vi "Interpolate and Measure.vi"(8 "error in (no error)":errorcluster, 9 "search results":cluster{"level":dbl, "value":dbl}[](array[cluster]), 10 "frequency (Hz)":dbl, 11 "measurement configuration":T2 {"acq sampling rate" format="%0.2f"; "master clock rate" format="%#_6pHz"; "frame clock rate" format="%#_6pHz"}) -> (0 "error out":errorcluster, 1 "spectrum":cluster{"x0":dbl, "dx":dbl, "magnitude":dbl[]}, 2 "time domain":waveform(dbl), 3 "results":T1, 4 "output power":dbl)   [LabVIEW 2021]
uses:
  Measurement Configuration.ctl
  shared/controls/digital audio protocol/data justification.ctl
  shared/controls/digital audio protocol/endianness.ctl
  shared/controls/digital audio protocol/digital edge.ctl
  shared/controls/digital audio protocol/logic level.ctl
  shared/controls/digital output level units.ctl
  shared/controls/weighting filter.ctl
  shared/controls/highpass filter.ctl
  shared/controls/lowpass filter.ctl
  shared/controls/sweep profile.ctl
  shared/controls/units - snr.ctl
  shared/controls/units - ratio.ctl
  shared/controls/regulation target.ctl
  shared/controls/regulation target value units.ctl
  Stepped Frequency Sweep_Class D Amplifier.lvlib
  <vilib>/Analysis/NI_AALPro.lvlib
  shared/controls/audio controls.lvlib
  shared/controls/single tone audio measurements.ctl
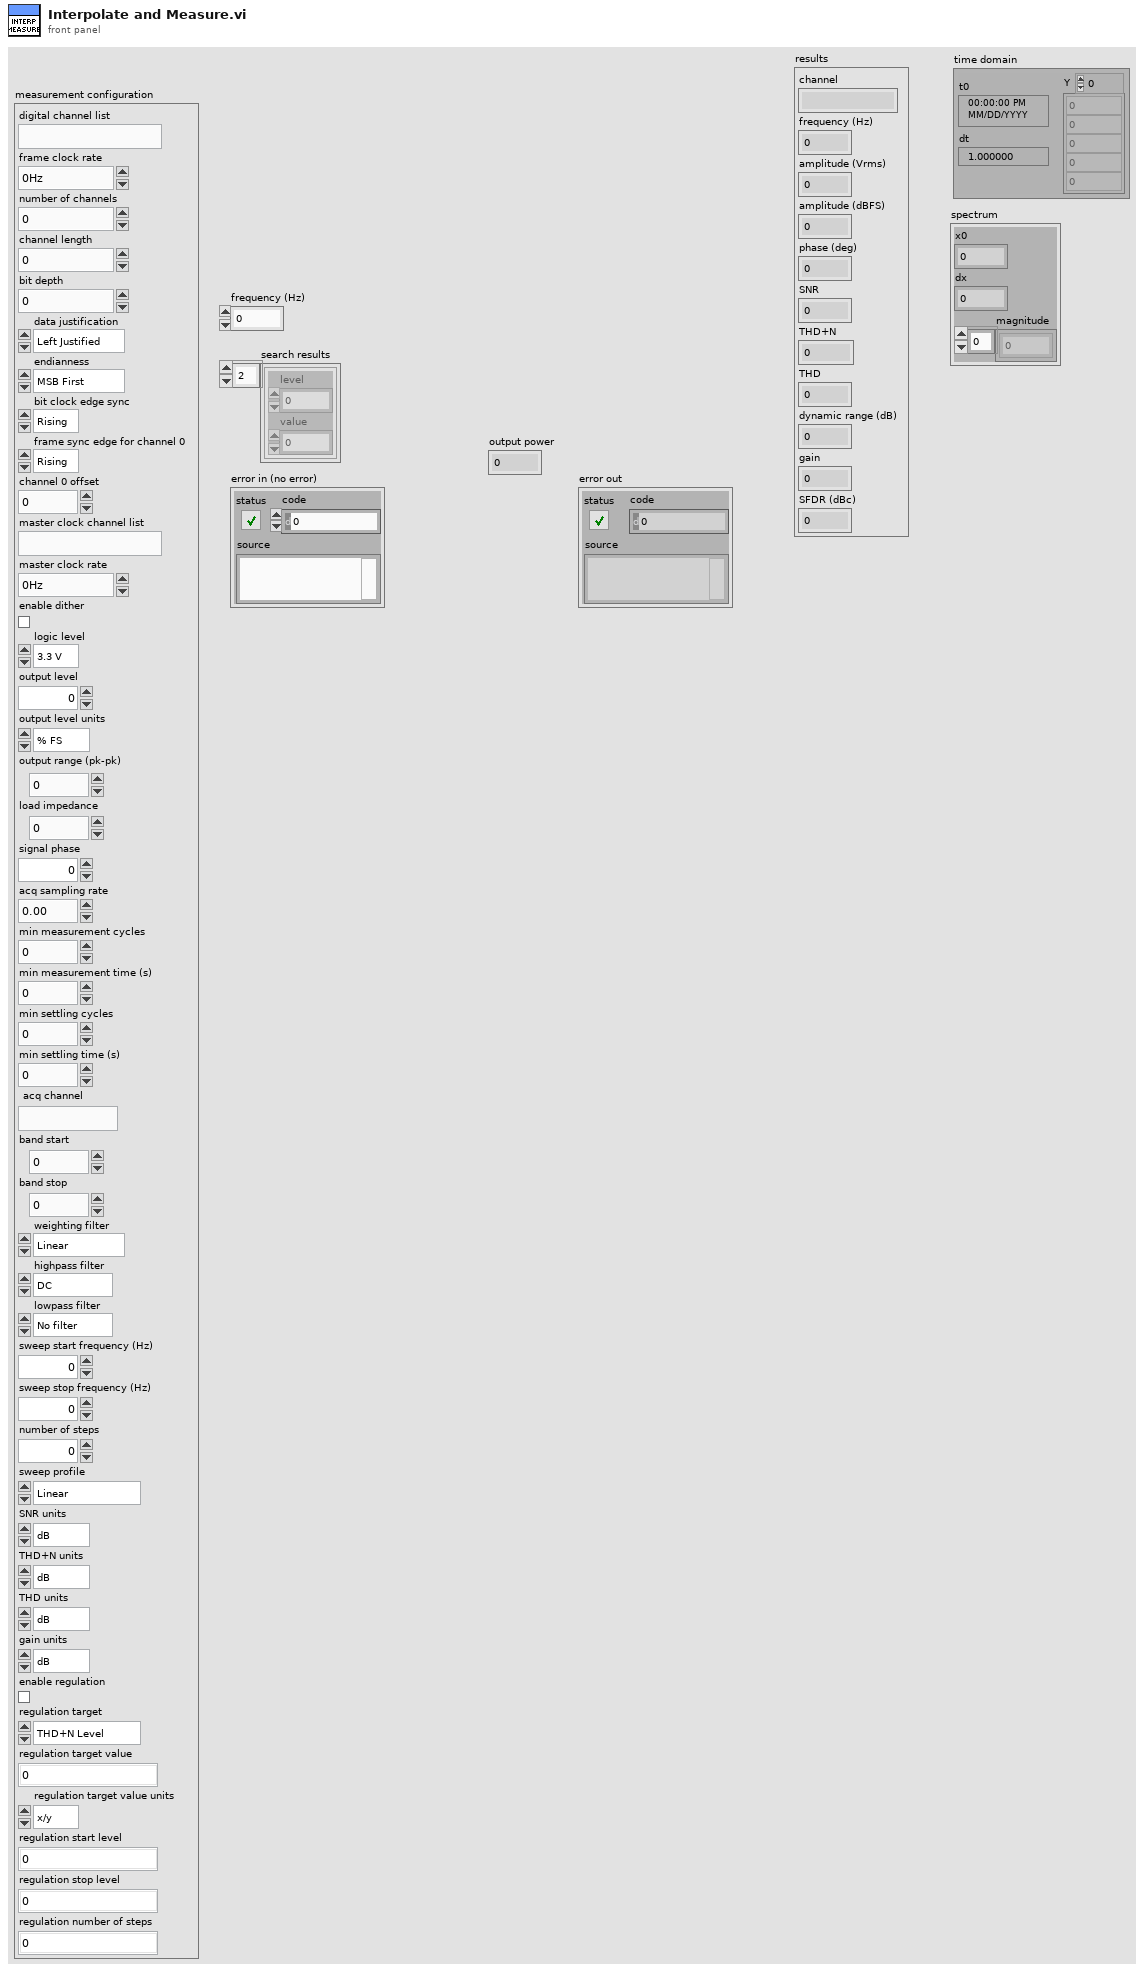
[diagram p1: front panel]
types:
  T1 = typedef "audio controls.lvlib/single tone audio measurements.ctl" = cluster{"channel":string, "frequency (Hz)":dbl, "amplitude (Vrms)":dbl, "amplitude (dBFS)":dbl, "phase (deg)":dbl, "SNR":dbl, "THD+N":dbl, "THD":dbl, "dynamic range (dB)":dbl, "gain":dbl, "SFDR (dBc)":dbl}
  T2 = typedef "Stepped Frequency Sweep_Class D Amplifier.lvlib/Measurement Configuration.ctl" = cluster{"digital channel list":string, "frame clock rate":dbl, "number of channels":u32, "channel length":u32, "bit depth":u32, "data justification":T3, "endianness":T4, "bit clock edge sync":T5, "frame sync edge for channel 0":T5, "channel 0 offset":u32, "master clock channel list":string, "master clock rate":dbl, "enable dither":bool, "logic level":T6, "output level":dbl, "output level units":T7, "output range (pk-pk)":dbl, "load impedance":dbl, "signal phase":dbl, "acq sampling rate":dbl, "min measurement cycles":u32, "min measurement time (s)":dbl, "min settling cycles":u32, "min settling time (s)":dbl, "acq channel":string, "band start":dbl, "band stop":dbl, "weighting filter":T8, "highpass filter":T9, "lowpass filter":T10, "sweep start frequency (Hz)":dbl, "sweep stop frequency (Hz)":dbl, "number of steps":u32, "sweep profile":T11, "SNR units":T12, "THD+N units":T13, "THD units":T13, "gain units":T13, "enable regulation":bool, "regulation target":T14, "regulation target value":dbl, "regulation target value units":T15, "regulation start level":dbl, "regulation stop level":dbl, "regulation number of steps":u32}
  T3 = typedef "data justification.ctl" = enum32{"Left Justified", "Right Justified"}
  T4 = typedef "endianness.ctl" = enum32{"MSB First", "LSB First"}
  T5 = typedef "digital edge.ctl" = enum32{"Rising", "Falling"}
  T6 = typedef "logic level.ctl" = enum32{"3.3 V", "1.8 V", "1.2 V"}
  T7 = typedef "audio controls.lvlib/digital output level units.ctl" = enum32{"% FS", "dBFS"}
  T8 = typedef "weighting filter.ctl" = enum32{"Linear", "A-weighting", "B-weighting", "C-weighting"}
  T9 = typedef "highpass filter.ctl" = enum32{"DC", "AC"}
  T10 = typedef "lowpass filter.ctl" = enum32{"No filter", "AES17 20kHz", "AES17 40kHz"}
  T11 = typedef "audio controls.lvlib/sweep profile.ctl" = enum32{"Linear", "Logarithmic"}
  T12 = typedef "audio controls.lvlib/units - snr.ctl" = enum32{"dB", "x/y"}
  T13 = typedef "audio controls.lvlib/units - ratio.ctl" = enum32{"dB", "%", "x/y"}
  T14 = typedef "regulation target.ctl" = enum32{"THD+N Level", "THD+N Ratio", "RMS Level", "RMS Ratio", "Output Power"}
  T15 = typedef "regulation target value units.ctl" = enum32{"x/y", "%", "dB", "Vrms", "W"}
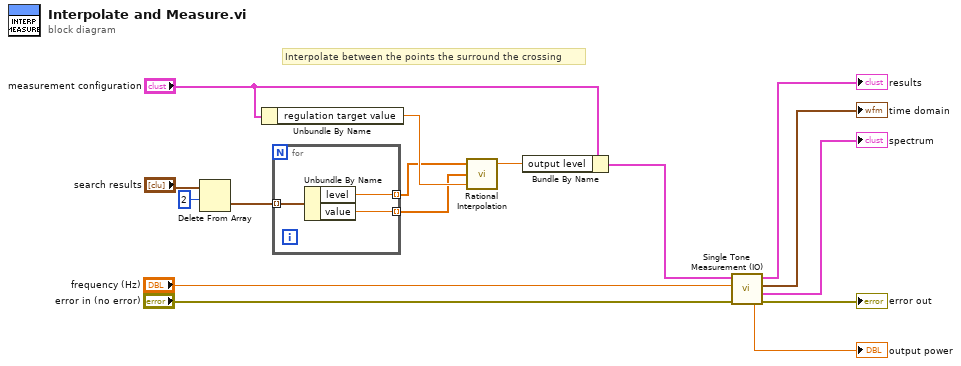
[diagram p0: block diagram]
diagram:
  # "Interpolate between the points the surround the crossing"
  n1 = Delete From Array(array="search results", length=2) -> (deleted portion=w10:cluster{"level":dbl, "value":dbl}[])  [unwired: 1 in, 1 out]
  n2 = Unbundle By Name("measurement configuration") -> ("regulation target value"=w8:dbl)
  n3 = for {
    tunnel: w10 -> [w19] mode=indexing
    tunnel: [w18] -> w7 mode=indexing
    tunnel: [w17] -> w6 mode=indexing
    n4 = Unbundle By Name(w19) -> ("level"=w17:dbl, "value"=w18:dbl)
  }
  n5 = call <vilib>:"Rational Interpolation.vi"("x value"=w8, "X"=w7, "Y"=w6) -> ("interpolation value"=w5:dbl)  [unwired: 2 out]
  n6 = Bundle By Name(cluster="measurement configuration", "output level"=w5) -> (w13:T2)
  n7 = call "Single Tone Measurement (IO).vi"("error in (no error)"="error in (no error)", "sweep start frequency (Hz)"="frequency (Hz)", "measurement configuration"=w13) -> ("error out"=→"error out":errorcluster, "spectrum"=→"spectrum":cluster{"x0":dbl, "dx":dbl, "magnitude":dbl[]}, "time domain"=→"time domain":waveform(dbl), "results"=→"results":T1, "output power"=→"output power":dbl)  [unwired: 4 in]
